vi "Calculate_Row_Time.vi"(2 "Row Start Time (Sec Since 1904)":dbl, 3 "Multi Run Row":T1 {"Row Duration (mins)" format="%#.1f"; "Row No" min=0; "Trace Gas Concentration (%)" min=0.0 format="%#.2f"; "Emission Rate (l/min)" format="%#.2f"; "Tunnel Speed" format="%#.2f"; "Start X" format="%#.2f"; "Start Y" format="%#.2f"; "Start Z" format="%#.2f"; "End X" format="%#.2f"; "End Y" format="%#.2f"; "End Z" format="%#.2f"; "Averaging time (min)" min=0.0 format="%#.2f"}) -> (0 "Scalable Time (Sec)":dbl format="%.2f", 1 "Fixed Time (Sec)":dbl format="%.2f")   [LabVIEW 2012]
uses:
  Traverse_cluster.ctl
  Spacing.ctl
  Controls/Multi_run_mode.ctl
  Globals/Preference_global.vi
  Globals/Extra_Commands_Global.vi
panel:
  # "X           Y            Z"
  # "Start"
  # "End"
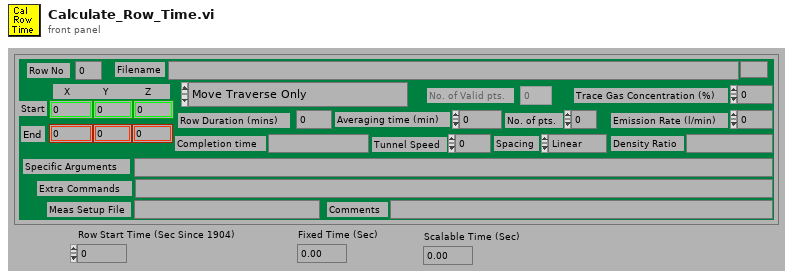
[diagram p1: front panel]
types:
  T1 = typedef "Traverse_cluster.ctl" = cluster{"Start X":dbl, "Start Y":dbl, "Start Z":dbl, "End X":dbl, "End Y":dbl, "End Z":dbl, "No. of pts.":i32, "Spacing":T2, "Filename":path, "Tunnel Speed":dbl, "Averaging time (min)":dbl, "Extra Commands":string, "Specific Arguments":string, "Emission Rate (l/min)":dbl, "Trace Gas Concentration (%)":dbl, "Density Ratio":string, "Comments":string, "Row No":i32, "Row Type Selector":T3, "Completion time":string, "Row Duration (mins)":dbl, "No. of Valid pts.":i32, "Meas Setup File":string}
  T2 = typedef "Spacing.ctl" = enum16{"Linear", "Log", "Gauss", "Specified", "N/A"}
  T3 = typedef "Multi_run_mode.ctl" = enum16{"Move Traverse Only", "Set Tunnel Speed Only", "Set Source Only", "Set Measurement Conditions", "Single Measurement", "Vertical Profile", "Lateral Profile", "Longitudinal Profile", "Explore Volume", "Multi-Axis Profile", "Auto Calibrate", "Meas Fast FID Bkgnd", "Check Beam Power", "Scanning Valve Measurement", "Run VI Named:", "Set ADAM Ch", "Wait (minutes)", "Send Message", "Synchronize With:", "Fall Back to this Row", "Turn Off Row Repeating", "Blank Row", "Traverse 3D Volume"}
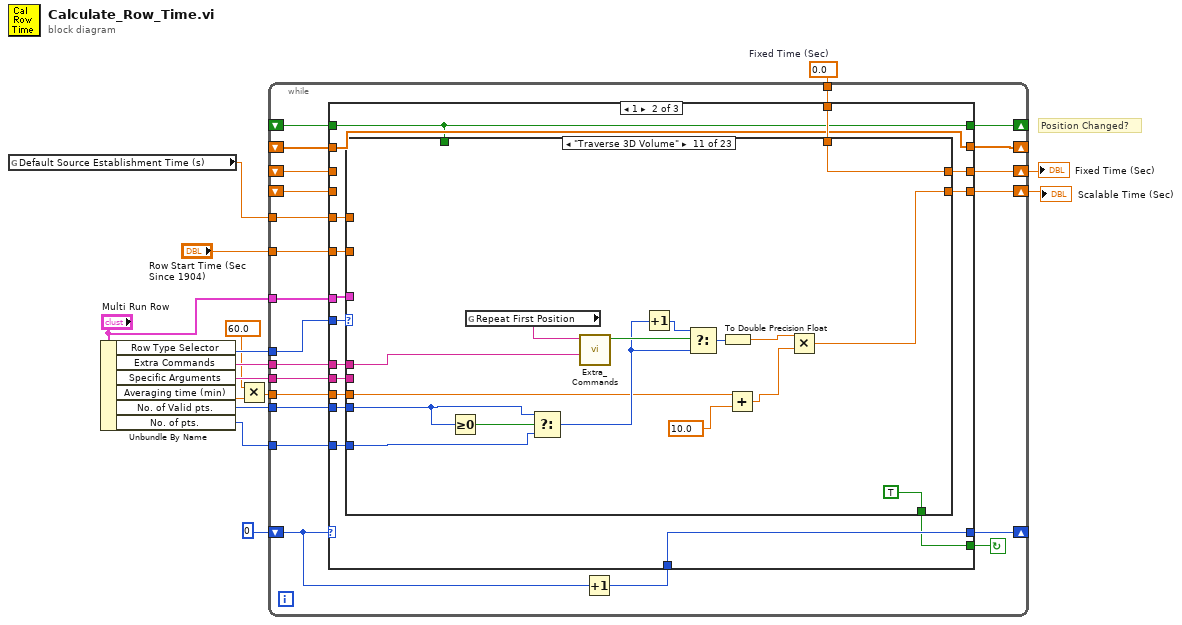
[diagram p0: block diagram]
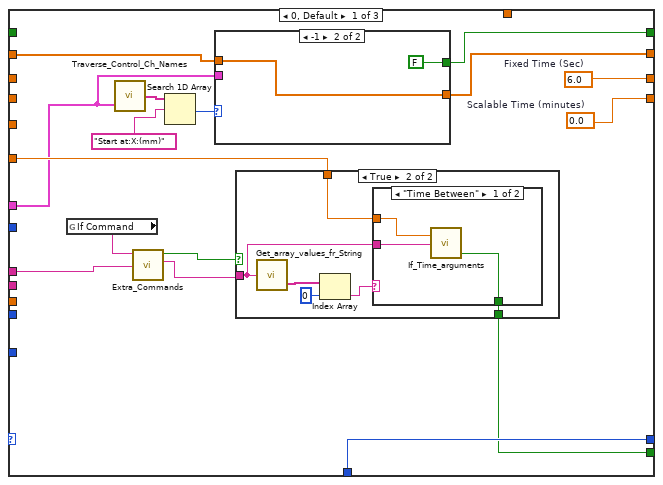
[diagram p2: hidden frame]
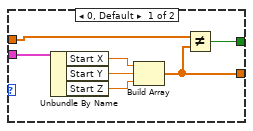
[diagram p3: hidden frame]
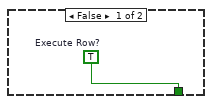
[diagram p4: hidden frame]
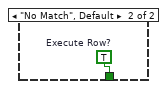
[diagram p5: hidden frame]
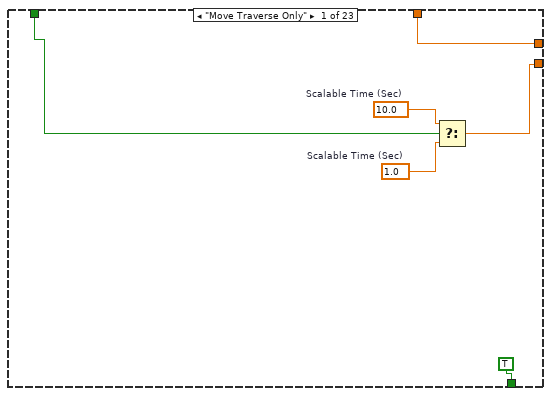
[diagram p6: hidden frame]
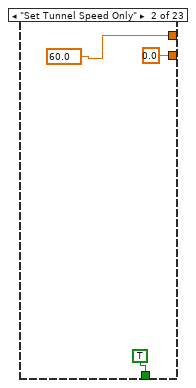
[diagram p7: hidden frame]
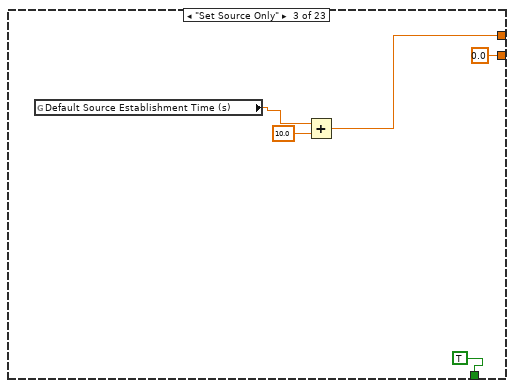
[diagram p8: hidden frame]
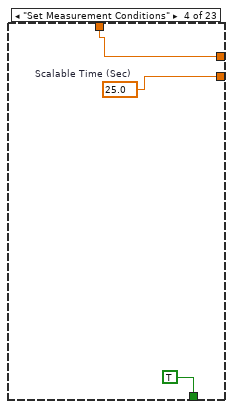
[diagram p9: hidden frame]
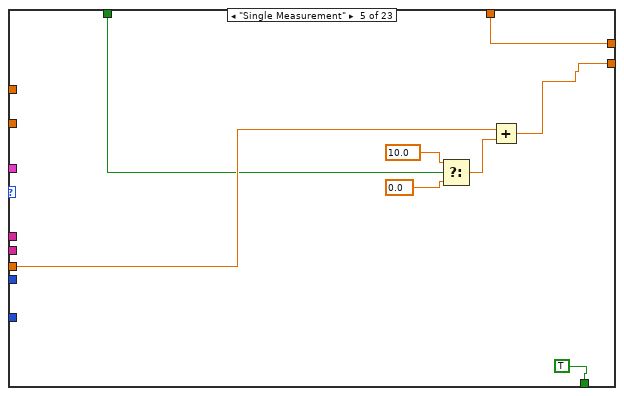
[diagram p10: hidden frame]
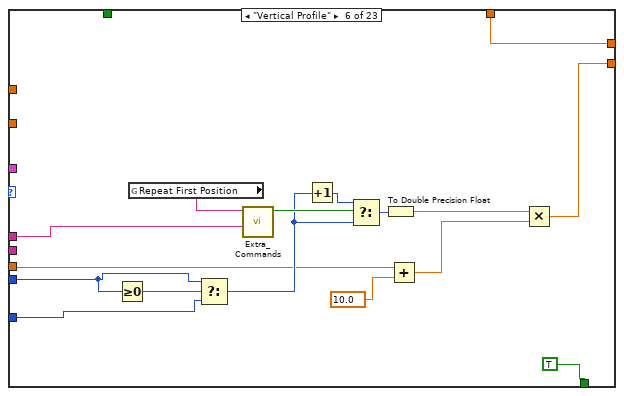
[diagram p11: hidden frame]
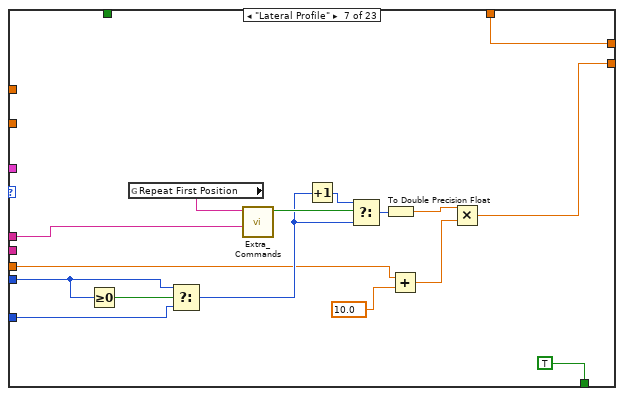
[diagram p12: hidden frame]
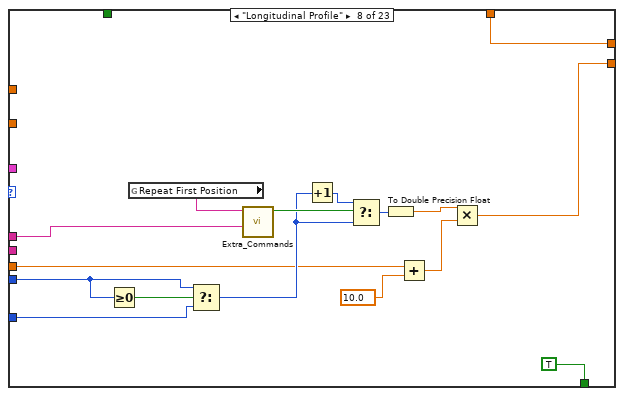
[diagram p13: hidden frame]
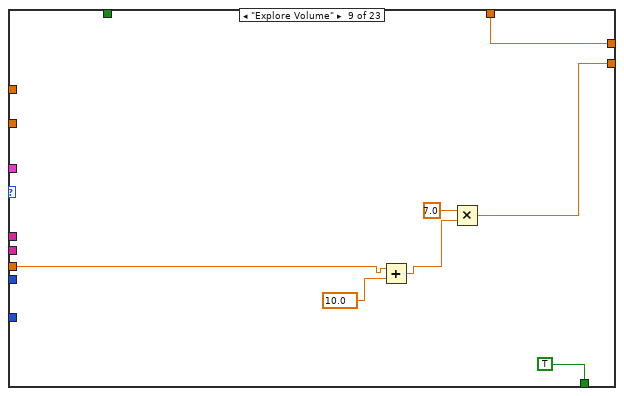
[diagram p14: hidden frame]
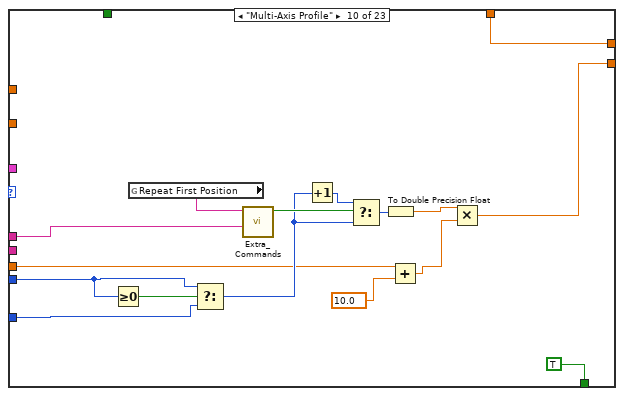
[diagram p15: hidden frame]
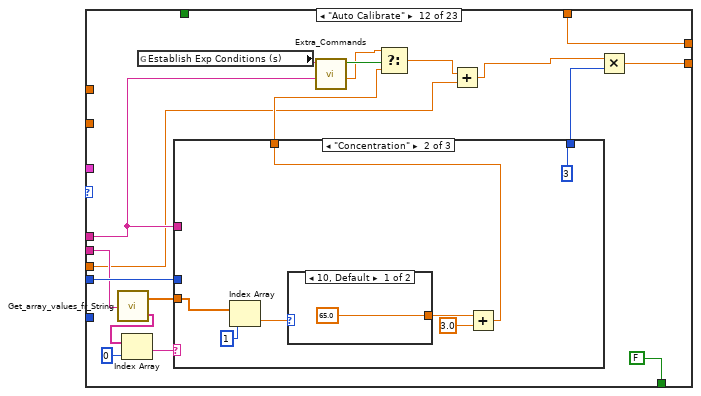
[diagram p16: hidden frame]
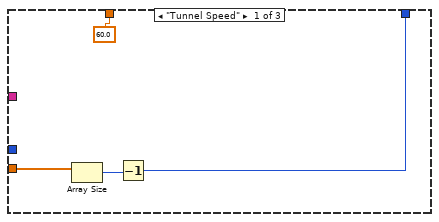
[diagram p17: hidden frame]
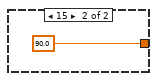
[diagram p18: hidden frame]
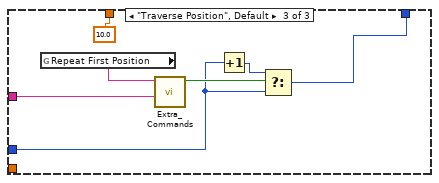
[diagram p19: hidden frame]
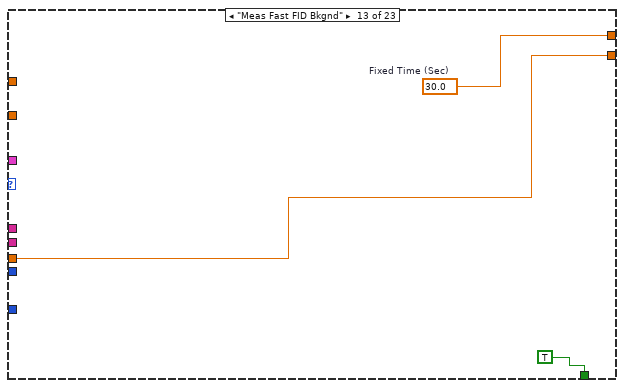
[diagram p20: hidden frame]
diagram:
  w4 = 0.0  # Fixed Time (Sec)
  # "Position Changed?"
  n1 = global read "Preference_global.vi" "Default Source Establishment Time (s)"() -> (w1:dbl)
  n2 = Unbundle By Name("Multi Run Row") -> ("Row Type Selector"=w10:T3, "Extra Commands"=w14:string, "Specific Arguments"=w8:string, "Averaging time (min)"=w7:dbl, "No. of Valid pts."=w9:i32, "No. of pts."=w3:i32)
  n3 = Multiply(x=60.0, y=w7) -> (x*y=w5:dbl)
  n4 = while {
    tunnel: w4 -> [w23]
    tunnel: w8 -> [w26]
    tunnel: w9 -> [w27]
    tunnel: w5 -> [w28]
    tunnel: w10 -> [w29]
    tunnel: "Row Start Time (Sec Since 1904)" -> [w32]
    tunnel: w14 -> [w33]
    shift-left: _ -> [w25]
    shift-right: [w30] -> w12
    shift-left: _ -> [w24]
    shift-right: [w31] -> w11
    shift-left: 0 -> [w36]
    shift-right: [w34] -> _
    tunnel: w3 -> [w22]
    tunnel: "Multi Run Row" -> [w21]
    shift-right: [w20] -> _
    shift-left: _ -> [w19]
    shift-right: [w18] -> _
    shift-left: _ -> [w17]
    tunnel: w1 -> [w16]
    stop <- w37 continue-if-true
    n5 = Increment(x=w36) -> (x+1=w35:i32)
    n6 = case shown="1" w36 {
      tunnel: [w48 w79 FALSE ("Execute Row?")] -> w37
      tunnel: w35 -> [w53 w88 w286]
      tunnel: [w53 w88 w286] -> w34
      tunnel: w33 -> [w49 w84 w291]
      tunnel: w32 -> [w47 w81 _]
      tunnel: [w46 w87 w288] -> w31
      tunnel: [w45 w86 w293] -> w30
      tunnel: w29 -> [_ w89 _]
      tunnel: w28 -> [_ w85 _]
      tunnel: w27 -> [_ w83 _]
      tunnel: w26 -> [_ w82 _]
      tunnel: w25 -> [_ _ w293]
      tunnel: w24 -> [_ _ w289]
      tunnel: w23 -> [_ w80 _]
      tunnel: w22 -> [_ w78 _]
      tunnel: w21 -> [w41 w74 _]
      tunnel: [w40 w77 w283] -> w20
      tunnel: w19 -> [w39 w77 w283]
      tunnel: [w38 w76 w284] -> w18
      tunnel: w17 -> [_ w76 w284]
      tunnel: w16 -> [_ w75 _]
      frame 0, Default {
        w46 = 6.0  # Fixed Time (Sec)
        w45 = 0.0  # Scalable Time (minutes)
        n7 = global read "Extra_Commands_Global.vi" "If Command"() -> (w51:string)
        n8 = call "Traverse_Control_Ch_Names.vi"("Traverse line"=w41) -> ("Channel names"=w44:string[])  [unwired: 1 in]
        n9 = call "Extra_Commands.vi"("String to Search"=w49, "Command"=w51) -> ("String Value"=w50:string, "Command Found"=w52:bool)  [unwired: 1 in, 3 out]
        n10 = Search 1D Array(1D array=w44, element="Start at:X:(mm)" ("Label for value")) -> (index of element=w42:i32)  [unwired: 1 out]
        n11 = case shown="-1" w42 {
          tunnel: w41 -> [w60 _]
          tunnel: [w56 w62] -> w40
          tunnel: w39 -> [w55 w62]
          tunnel: [w54 FALSE] -> w38
          frame 0, Default {
            n12 = Unbundle By Name(w60) -> ("Start X"=w59:dbl, "Start Y"=w58:dbl, "Start Z"=w57:dbl)
            n13 = Build Array(w59, w58, w57) -> (w56:dbl[])
            n14 = Not Equal?(x=w55, y=w56) -> (x != y?=w54:bool)
          }
          frame -1 {
          }
        }
        n15 = case shown="True" w52 {
          tunnel: w50 -> [_ w66]
          tunnel: [w63 w65] -> w48
          tunnel: w47 -> [_ w64]
          frame False {
            w63 = TRUE  # Execute Row?
          }
          frame True {
            n16 = call "Get_array_values_fr_String.vi"("String Value"=w66) -> ("String array"=w68:string[])  [unwired: 1 out]
            n17 = Index Array(array=w68, index=0 ("Index")) -> (element=w67:string)
            n18 = case shown="\"Time Between\"" w67 {
              tunnel: w66 -> [w72 _]
              tunnel: [w71 w73] -> w65
              tunnel: w64 -> [w70 _]
              frame "Time Between" {
                n19 = call "If_Time_arguments.vi"("seconds since 1Jan1904"=w70, "String Value"=w72) -> ("Execute Row?"=w71:bool)  [unwired: 2 out]
              }
              frame "No Match", Default {
                w73 = TRUE  # Execute Row?
              }
            }
          }
        }
      }
      frame 1 {
        n20 = case shown="\"Traverse 3D Volume\"" w89 {
          tunnel: [w95 60.0 ("Scalable Time (Sec)") w100 w105 w114 w123 w139 w156 w168 w178 w194 w209 w242 w244 w250 w251 w255 w263 w270 w273 w276 w279 w282] -> w87
          tunnel: [w90 0.0 0.0 w104 w108 w126 w142 w158 w169 w181 w197 w210 w241 100.0 w246 w253 w254 w268 w271 w274 w277 w280 w282] -> w86
          tunnel: w85 -> [_ _ _ _ w110 w116 w131 w148 w164 w171 w187 w204 w241 _ w247 _ _ _ _ _ _ _ _]
          tunnel: w84 -> [_ _ _ _ _ w129 w145 w161 _ w184 w200 w213 _ _ _ _ _ _ _ _ _ _ _]
          tunnel: w83 -> [_ _ _ _ _ w120 w135 w151 _ w174 w190 w219 _ _ _ _ _ _ _ _ _ _ _]
          tunnel: w82 -> [_ _ _ _ _ _ _ _ _ _ _ w216 _ _ _ _ w259 w267 _ _ _ _ _]
          tunnel: w81 -> [_ _ _ _ _ _ _ _ _ _ _ _ _ _ _ _ _ w266 _ _ _ _ _]
          tunnel: w80 -> [w95 _ _ w105 w114 w123 w139 w156 w168 w178 w194 w209 _ w244 w250 w251 _ _ w270 w273 w276 w279 w282]
          tunnel: [TRUE TRUE TRUE TRUE TRUE TRUE TRUE TRUE TRUE TRUE TRUE FALSE TRUE TRUE TRUE TRUE TRUE FALSE TRUE TRUE FALSE FALSE FALSE] -> w79
          tunnel: w78 -> [_ _ _ _ _ w119 w134 w152 _ w175 w191 _ _ _ _ _ _ _ _ _ _ _ _]
          tunnel: w76 -> [w93 _ _ _ w107 _ _ _ _ _ _ _ _ _ _ _ _ _ _ _ _ _ _]
          tunnel: w75 -> [_ _ _ _ _ _ _ _ _ _ _ _ _ _ _ _ _ _ _ _ _ _ _]
          tunnel: w74 -> [_ _ _ _ _ _ _ _ _ _ _ _ _ _ _ _ w256 _ _ _ _ _ _]
          frame "Move Traverse Only" {
            w91 = 1.0  # Scalable Time (Sec)
            w92 = 10.0  # Scalable Time (Sec)
            n21 = Select(t=w92, s=w93, f=w91) -> (s? t:f=w90:dbl)
          }
          frame "Set Tunnel Speed Only" {
          }
          frame "Set Source Only" {
            n22 = global read "Preference_global.vi" "Default Source Establishment Time (s)"() -> (w102:dbl)
            n23 = Add(x=w102, y=10.0) -> (x+y=w100:dbl)
          }
          frame "Set Measurement Conditions" {
            w104 = 25.0  # Scalable Time (Sec)
          }
          frame "Single Measurement" {
            n24 = Select(t=10.0 ("Scalable Time (Sec)"), s=w107, f=0.0 ("Scalable Time (Sec)")) -> (s? t:f=w109:dbl)
            n25 = Add(x=w110, y=w109) -> (x+y=w108:dbl)
          }
          frame "Vertical Profile" {
            n26 = Greater Or Equal To 0?(x=w120) -> (x >= 0?=w121:bool)
            n27 = global read "Extra_Commands_Global.vi" "Repeat First Position"() -> (w130:string)
            n28 = Select(t=w120, s=w121, f=w119) -> (s? t:f=w118:i32)
            n29 = call "Extra_Commands.vi"("String to Search"=w129, "Command"=w130) -> ("Command Found"=w128:bool)  [unwired: 1 in, 4 out]
            n30 = Increment(x=w118) -> (x+1=w127:i32)
            n31 = Select(t=w127, s=w128, f=w118) -> (s? t:f=w125:i32)
            n32 = To Double Precision Float(number=w125) -> (double precision float=w124:dbl)
            n33 = Add(x=w116, y=10.0 ("Scalable Time (Sec)")) -> (x+y=w115:dbl)
            n34 = Multiply(x=w124, y=w115) -> (x*y=w126:dbl)
          }
          frame "Lateral Profile" {
            n35 = Greater Or Equal To 0?(x=w135) -> (x >= 0?=w137:bool)
            n36 = global read "Extra_Commands_Global.vi" "Repeat First Position"() -> (w146:string)
            n37 = Select(t=w135, s=w137, f=w134) -> (s? t:f=w136:i32)
            n38 = call "Extra_Commands.vi"("String to Search"=w145, "Command"=w146) -> ("Command Found"=w144:bool)  [unwired: 1 in, 4 out]
            n39 = Increment(x=w136) -> (x+1=w143:i32)
            n40 = Select(t=w143, s=w144, f=w136) -> (s? t:f=w141:i32)
            n41 = To Double Precision Float(number=w141) -> (double precision float=w140:dbl)
            n42 = Add(x=w131, y=10.0 ("Scalable Time (Sec)")) -> (x+y=w132:dbl)
            n43 = Multiply(x=w140, y=w132) -> (x*y=w142:dbl)
          }
          frame "Longitudinal Profile" {
            n44 = Greater Or Equal To 0?(x=w151) -> (x >= 0?=w153:bool)
            n45 = global read "Extra_Commands_Global.vi" "Repeat First Position"() -> (w162:string)
            n46 = Select(t=w151, s=w153, f=w152) -> (s? t:f=w150:i32)
            n47 = call "Extra_Commands.vi"("String to Search"=w161, "Command"=w162) -> ("Command Found"=w160:bool)  [unwired: 1 in, 4 out]
            n48 = Increment(x=w150) -> (x+1=w159:i32)
            n49 = Select(t=w159, s=w160, f=w150) -> (s? t:f=w157:i32)
            n50 = To Double Precision Float(number=w157) -> (double precision float=w155:dbl)
            n51 = Add(x=w148, y=10.0 ("Scalable Time (Sec)")) -> (x+y=w147:dbl)
            n52 = Multiply(x=w155, y=w147) -> (x*y=w158:dbl)
          }
          frame "Explore Volume" {
            n53 = Add(x=w164, y=10.0 ("Scalable Time (Sec)")) -> (x+y=w163:dbl)
            n54 = Multiply(x=7.0, y=w163) -> (x*y=w169:dbl)
          }
          frame "Multi-Axis Profile" {
            n55 = Greater Or Equal To 0?(x=w174) -> (x >= 0?=w176:bool)
            n56 = global read "Extra_Commands_Global.vi" "Repeat First Position"() -> (w185:string)
            n57 = Select(t=w174, s=w176, f=w175) -> (s? t:f=w173:i32)
            n58 = call "Extra_Commands.vi"("String to Search"=w184, "Command"=w185) -> ("Command Found"=w183:bool)  [unwired: 1 in, 4 out]
            n59 = Increment(x=w173) -> (x+1=w182:i32)
            n60 = Select(t=w182, s=w183, f=w173) -> (s? t:f=w180:i32)
            n61 = To Double Precision Float(number=w180) -> (double precision float=w179:dbl)
            n62 = Add(x=w171, y=10.0 ("Scalable Time (Sec)")) -> (x+y=w170:dbl)
            n63 = Multiply(x=w179, y=w170) -> (x*y=w181:dbl)
          }
          frame "Traverse 3D Volume" {
            n64 = Greater Or Equal To 0?(x=w190) -> (x >= 0?=w192:bool)
            n65 = global read "Extra_Commands_Global.vi" "Repeat First Position"() -> (w201:string)
            n66 = Select(t=w190, s=w192, f=w191) -> (s? t:f=w189:i32)
            n67 = call "Extra_Commands.vi"("String to Search"=w200, "Command"=w201) -> ("Command Found"=w199:bool)  [unwired: 1 in, 4 out]
            n68 = Increment(x=w189) -> (x+1=w198:i32)
            n69 = Select(t=w198, s=w199, f=w189) -> (s? t:f=w196:i32)
            n70 = To Double Precision Float(number=w196) -> (double precision float=w195:dbl)
            n71 = Add(x=w187, y=10.0 ("Scalable Time (Sec)")) -> (x+y=w186:dbl)
            n72 = Multiply(x=w195, y=w186) -> (x*y=w197:dbl)
          }
          frame "Auto Calibrate" {
            n73 = call "Get_array_values_fr_String.vi"("String Value"=w216) -> ("Numeric Array"=w212:dbl[], "String array"=w218:string[])
            n74 = Index Array(array=w218, index=0 ("Index")) -> (element=w215:string)
            n75 = global read "Extra_Commands_Global.vi" "Establish Exp Conditions (s)"() -> (w214:string)
            n76 = case shown="\"Concentration\"" w215 {
              tunnel: w213 -> [_ _ w238]
              tunnel: w219 -> [_ _ w236]
              tunnel: [w221 3 ("No. of pts.") w234] -> w211
              tunnel: w212 -> [w223 w228 _]
              tunnel: [60.0 w224 10.0] -> w206
              frame "Tunnel Speed" {
                n77 = Array Size(array=w223) -> (size(s)=w222:i32)
                n78 = Decrement(x=w222) -> (x-1=w221:i32)
              }
              frame "Concentration" {
                n79 = Index Array(array=w228, index=1) -> (element=w227:dbl)
                n80 = case shown="10, Default" w227 {
                  tunnel: [65.0 ("Seconds to wait") 90.0 ("Seconds to wait")] -> w226
                  frame 10, Default {
                  }
                  frame 15 {
                  }
                }
                n81 = Add(x=w226, y=3.0) -> (x+y=w224:dbl)
              }
              frame "Traverse Position", Default {
                n82 = global read "Extra_Commands_Global.vi" "Repeat First Position"() -> (w239:string)
                n83 = call "Extra_Commands.vi"("String to Search"=w238, "Command"=w239) -> ("Command Found"=w237:bool)  [unwired: 1 in, 4 out]
                n84 = Increment(x=w236) -> (x+1=w235:i32)
                n85 = Select(t=w235, s=w237, f=w236) -> (s? t:f=w234:i32)
              }
            }
            n86 = call "Extra_Commands.vi"("String to Search"=w213, "Command"=w214) -> ("Numeric Value"=w207:dbl, "Command Found"=w208:bool)  [unwired: 1 in, 3 out]
            n87 = Select(t=w207, s=w208, f=w206) -> (s? t:f=w205:dbl)
            n88 = Add(x=w205, y=w204) -> (x+y=w203:dbl)
            n89 = Multiply(x=w203, y=w211) -> (x*y=w210:dbl)
          }
          frame "Meas Fast FID Bkgnd" {
            w242 = 30.0  # Fixed Time (Sec)
          }
          frame "Check Beam Power" {
          }
          frame "Scanning Valve Measurement" {
            n90 = Add(x=w247, y=5.0 ("Scalable Time (Sec)")) -> (x+y=w246:dbl)
          }
          frame "Set ADAM Ch" {
            w253 = 5.0  # Scalable Time (Sec)
          }
          frame "Run VI Named:" {
            n91 = Match Pattern(string=w259, regular expression=";") -> (before substring=w258:string)  [unwired: 4 out]
            n92 = call <vilib>:"Trim Whitespace.vi"("string"=w258) -> ("trimmed string"=w257:string)  [unwired: 1 in]
            n93 = call "Run_VI_Named_specific.vi"("Run VI Named String"=w257, "Multi Run Row"=w256) -> ("Scalable Time (Sec)"=w254:dbl, "Fixed Time (Sec)"=w255:dbl)  [unwired: 8 out]
          }
          frame "Wait (minutes)" {
            w268 = 0.0  # Scalable Time (Sec)
            n94 = call "Wait_Case_Arg.vi"("Specific Argument"=w267, "seconds since 1Jan1904"=w266) -> ("Minutes To Wait"=w265:dbl)  [unwired: 4 out]
            n95 = Multiply(x=w265, y=60.0) -> (x*y=w263:dbl)
          }
          frame "Send Message" {
            w271 = 1.0  # Scalable Time (Sec)
          }
          frame "Synchronize With:" {
            w274 = 30.0  # Scalable Time (Sec)
          }
          frame "Fall Back to this Row" {
            w277 = 2.0  # Scalable Time (Sec)
          }
          frame "Turn Off Row Repeating" {
            w280 = 10.0  # Scalable Time (Sec)
          }
          frame "Blank Row" {
          }
        }
      }
      frame 2 {
        n96 = global read "Extra_Commands_Global.vi" "Establish Exp Conditions (s)"() -> (w292:string)
        n97 = call "Extra_Commands.vi"("String to Search"=w291, "Command"=w292) -> ("Numeric Value"=w290:dbl, "Command Found"=w287:bool)  [unwired: 1 in, 3 out]
        n98 = case shown="True" w287 {
          tunnel: w290 -> [_ w295]
          tunnel: w289 -> [w294 w297]
          tunnel: [w294 w296] -> w288
          frame False {
          }
          frame True {
            n99 = Add(x=w297, y=w295) -> (x+y=w296:dbl)
          }
        }
      }
    }
  }
  "Fixed Time (Sec)" <- w11
  "Scalable Time (Sec)" <- w12
